vi "Write Experiment info.vi"(8 "error in (no error)":errorcluster, 10 "Experiment info":T1={"attendee"=[], "title"="", "magnet_System"="", "proposal_Number"="", "proposal_Title"="Undocumented activity", "facility"="", "pi"="", "dtstart"="", "dtend"="", "dtstamp"="", "location"="", "summary"="", "pid"="Undocumented", "support"="", "uid"="", "start"=0, "id"=0}, 11 "Log Record in":refnum<class "Log Record.lvclass">) -> (0 "error out":errorcluster, 3 "Log Record out":refnum<class "Log Record.lvclass">)   [LabVIEW 2024, in "Log Record.lvclass"]
uses:
  Log Record.lvclass
  Log Record.lvclass/Log Record.ctl
  NHMFL_Core/Libraries/FAIR Data/MagX/Experiment info.ctl
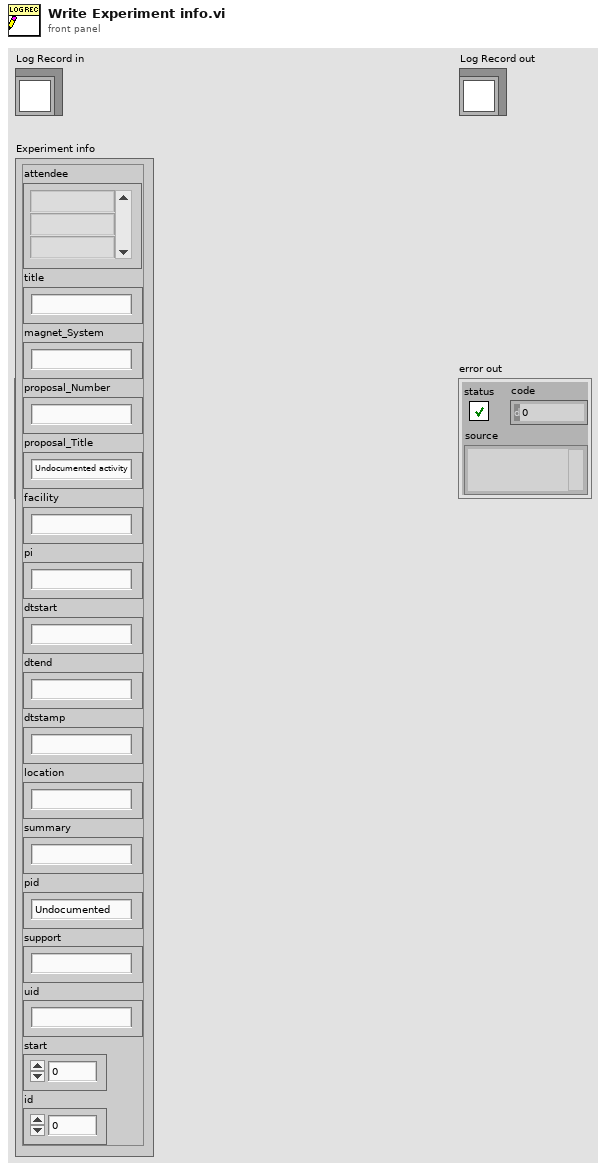
[diagram p1: front panel]
types:
  T1 = typedef "Experiment info.ctl" = cluster{"attendee":string[], "title":string, "magnet_System":string, "proposal_Number":string, "proposal_Title":string, "facility":string, "pi":string, "dtstart":string, "dtend":string, "dtstamp":string, "location":string, "summary":string, "pid":string, "support":string, "uid":string, "start":u64, "id":u64}
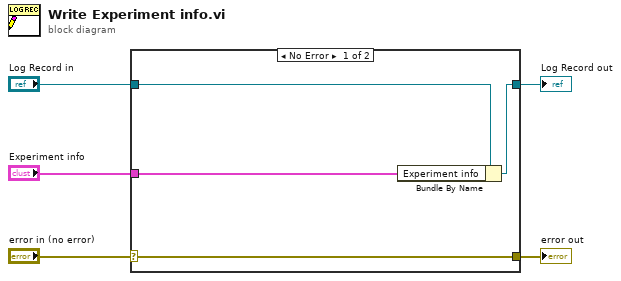
[diagram p0: block diagram]
diagram:
  n1 = case shown="No Error" "error in (no error)" {
    selector: "error in (no error)" -> [w9 w10]
    tunnel: [w9 w10] -> w4
    tunnel: [w7 w11] -> w2
    tunnel: "Log Record in" -> [w8 w11]
    tunnel: "Experiment info" -> [w6 _]
    frame No Error {
      n2 = Bundle By Name(cluster=w8, "Experiment info"=w6) -> (w7:refnum<class "Log Record.lvclass">)
    }
    frame Error {
    }
  }
  "error out" <- w4
  "Log Record out" <- w2
